vi "DataPacker_PeriodicTasks.vi"(8 "error in (no error)":errorcluster) -> (0 "error out":errorcluster)   [LabVIEW 2018, in "feGEM DataPacker.lvlib"]
uses:
  feGEM DataPacker.lvlib
  1e514528-7480-4a8c-9df7-1b56009fffe7.vi
  1e514528-7480-4a8c-9df7-1b56009fffe7.vi/b07c45a3-98d6-488c-9a25-2d4bcfe6af64.vi
  <vilib>/Utility/SystemLogging/Write to System Log.vi
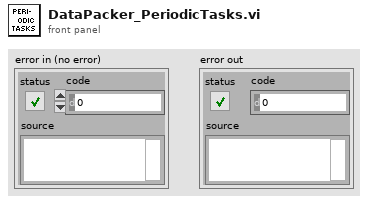
[diagram p1: front panel]
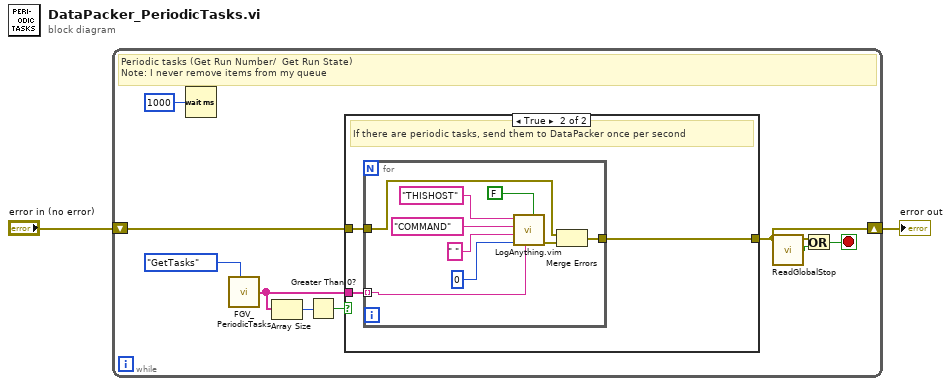
[diagram p0: block diagram]
diagram:
  n1 = while {
    shift-right: [w6] -> w2
    shift-left: "error in (no error)" -> [w7]
    stop <- w5 stop-if-true
    # "Periodic tasks (Get Run Number/  Get Run State)\nNote: I never remove items from my queue"
    n2 = Wait (ms)(milliseconds to wait=u32 1000) -> ()  [unwired: 1 out]
    n3 = call "FGV_PeriodicTasks.vi"("Task"=enum16{"AddTask", "GetTasks", "ClearTasks"}."GetTasks" ("Enum")) -> ("Tasks"=w8:string[])  [unwired: 4 in]
    n4 = Array Size(array=w8) -> (size(s)=w9:i32)
    n5 = Greater Than 0?(x=w9) -> (x > 0?=w10:bool)
    n6 = case shown="True" w10 {
      tunnel: w8 -> [_ w15]
      tunnel: w7 -> [w12 w14]
      tunnel: [w12 w13] -> w6
      frame False {
      }
      frame True {
        # "If there are periodic tasks, send them to DataPacker once per second"
        n7 = for {
          tunnel: w15 -> [w16] mode=indexing
          tunnel: w14 -> [w24]
          tunnel: [w23] -> w13
          n8 = call "LogAnything.vim"("Skip ODB on the way to \nhistories (fast, but no ALARMS possible)"=FALSE ("Get Default History Period from MIDAS\n(optional)"), "Equipment description (32 chars)"=w16, "Period to update history plots (seconds)\nUnset (65535) = Use MIDAS default in ODB\n0 = Record but do not put in histories"=0 ("Rate to update history plots"), "Array"=" ", "Variable Name"="COMMAND" ("Var Name"), "Category"="THISHOST") -> ("error out"=w19:errorcluster)  [unwired: 4 in, 1 out]
          n9 = Merge Errors(w24, w19) -> (w23:errorcluster)
        }
      }
    }
    n10 = call "ReadGlobalStop.vi"() -> ("Global DataPacker Stop"=w3:bool)
    n11 = Or(x=w6, y=w3) -> (x .or. y?=w5:bool)
  }
  "error out" <- w2
